vi "Autonomous Independent.vi"() -> ()   [LabVIEW 2014]
doc: "This VI is called when autonomous begins, and will automatically be terminated when autonomous ends. You can carry out timed or sensor driven robot movement independently without needing to return to the caller."
uses:
  <vilib>/Rock Robotics/WPI/Joystick/WPI_JoystickGetSetRefNum.vi
  <vilib>/Rock Robotics/Network Tables/SD Write Numeric Array.vi
  Robot Global Data.vi
  <vilib>/Rock Robotics/WPI/RobotDrive/WPI_RobotDriveGetSetRefNum.vi
  <vilib>/addons/control/pid/pid.llb/PID Advanced (DBL).vi
  <vilib>/Rock Robotics/WPI/RobotDrive/WPI_RobotDriveMecanumDrive_Cartesian.vi
  <vilib>/addons/control/pid/NI_PID_pid.lvlib
panel:
  out "distance":fxp<+/-,32,16>[](array[numeric])
  out "Current Movement, for debugging":T1 {"Z Joystick Value" scale=-1.0..1.0; "Y Joystick Value" scale=1.0..-1.0; "X Joystick Value" scale=-1.0..1.0}
  in  "Array of robot movements":T2(array[cluster]) {"Z Joystick Value" scale=-1.0..1.0; "Y Joystick Value" scale=1.0..-1.0; "X Joystick Value" scale=-1.0..1.0}
  # "Be sure to right-click and choose Data Operations>>Make Current Value default if you want to save the array values with the VI"
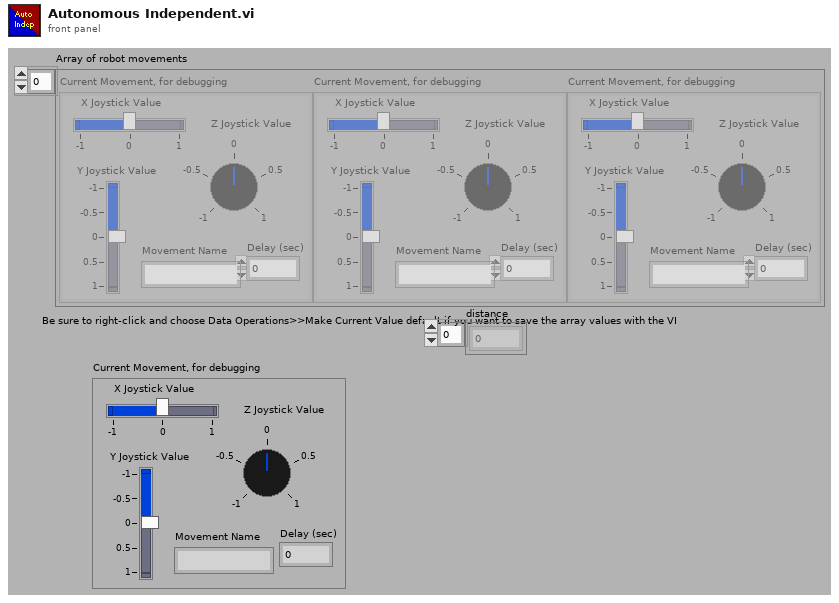
[diagram p1: front panel]
types:
  T1 = cluster{"X Joystick Value":dbl, "Y Joystick Value":dbl, "Z Joystick Value":dbl, "Delay (sec)":dbl, "Movement Name":string}
  T2 = cluster{"X Joystick Value":dbl, "Y Joystick Value":dbl, "Z Joystick Value":dbl, "Delay (sec)":dbl, "Movement Name":string}[]
  T3 = typedef "WPI_EncoderDevRef.ctl" = cluster{"DevStatus":errorcluster, "EncoderIndex":T4, "CounterIndex":T5, "DistancePerCount":dbl, "Decoding Type":T6}
  T4 = typedef "FPGA_EncoderIdx.ctl" = enum8{"Enc 0", "Enc 1", "Enc 2", "Enc 3", "Enc 4", "Enc 5", "Enc 6", "Enc 7", "Invalid"}
  T5 = typedef "FPGA_CounterCtrSystemIndex.ctl" = enum8{"Ctr 0", "Ctr 1", "Ctr 2", "Ctr 3", "Ctr 4", "Ctr 5", "Ctr 6", "Ctr 7", "Invalid"}
  T6 = typedef "WPI_EncoderType.ctl" = enum16{"1x", "2x", "4x"}
  T7 = typedef "WPI_RobotDriveDevRef.ctl" = cluster{"DevStatus":errorcluster, "Motors[]":T8[], "Square Inputs":bool, "Max Output":dbl}
  T8 = typedef "WPI_MotorControlDeviceRef.ctl" = cluster{"DeviceStatus":errorcluster, "Type":T9, "PWM":cluster{"Controller":T10, "PWM Channel":T11, "DeadBand":T12}, "CAN":cluster{"Device Number":u8, "Control Mode":T13, "Semaphore":T14, "Max Vout":dbl, "TalonSRX Control Mode":T15}, "Invert":bool, "TransformRef":T16, "InvTransformRef":T16}
  T9 = typedef "WPI_MotorControlType.ctl" = enum16{"PWM", "CAN", "CANTalonSRX"}
  T10 = typedef "FPGA_TypedefDigitalModule.ctl" = enum16{"Controller 1"}
  T11 = typedef "FPGA_DIOPWMChannel.ctl" = enum8{"PWM 0", "PWM 1", "PWM 2", "PWM 3", "PWM 4", "PWM 5", "PWM 6", "PWM 7", "PWM 8", "PWM 9", "PWM MXP 0", "PWM MXP 1", "PWM MXP 2", "PWM MXP 3", "PWM MXP 4", "PWM MXP 5", "PWM MXP 6", "PWM MXP 7", "PWM MXP 8", "PWM MXP 9", "Invalid"}
  T12 = typedef "WPI_PWMDeadband.ctl" = cluster{"Name":string, "maxPositivePwm":i32, "minPositivePwm":i32, "centerPwm":i32, "maxNegativePwm":i32, "minNegativePwm":i32, "angularRange":u16}
  T13 = typedef "WPI_CANJaguar_ControlMode.ctl" = enum8{"Percent VBus", "Current", "Speed", "Position", "Voltage"}
  T14 = typedef "Semaphore RefNum" = refnum<k1>
  T15 = typedef "WPI_CANTalonSRX_APIControlMode.ctl" = enum8{"Percent VBus", "Speed", "Position", "Slave", "Unchanged / Invalid"}
  T16 = typedef "WPI_PWMTransform_ConPane.ctl" = refnum<vi>
  T17 = typedef "WPI_JoystickDevRef.ctl" = cluster{"Device":T18}
  T18 = typedef "WPI_JoystickDeviceEnum.ctl" = enum16{"USB 0", "USB 1", "USB 2", "USB 3", "USB 4", "USB 5"}
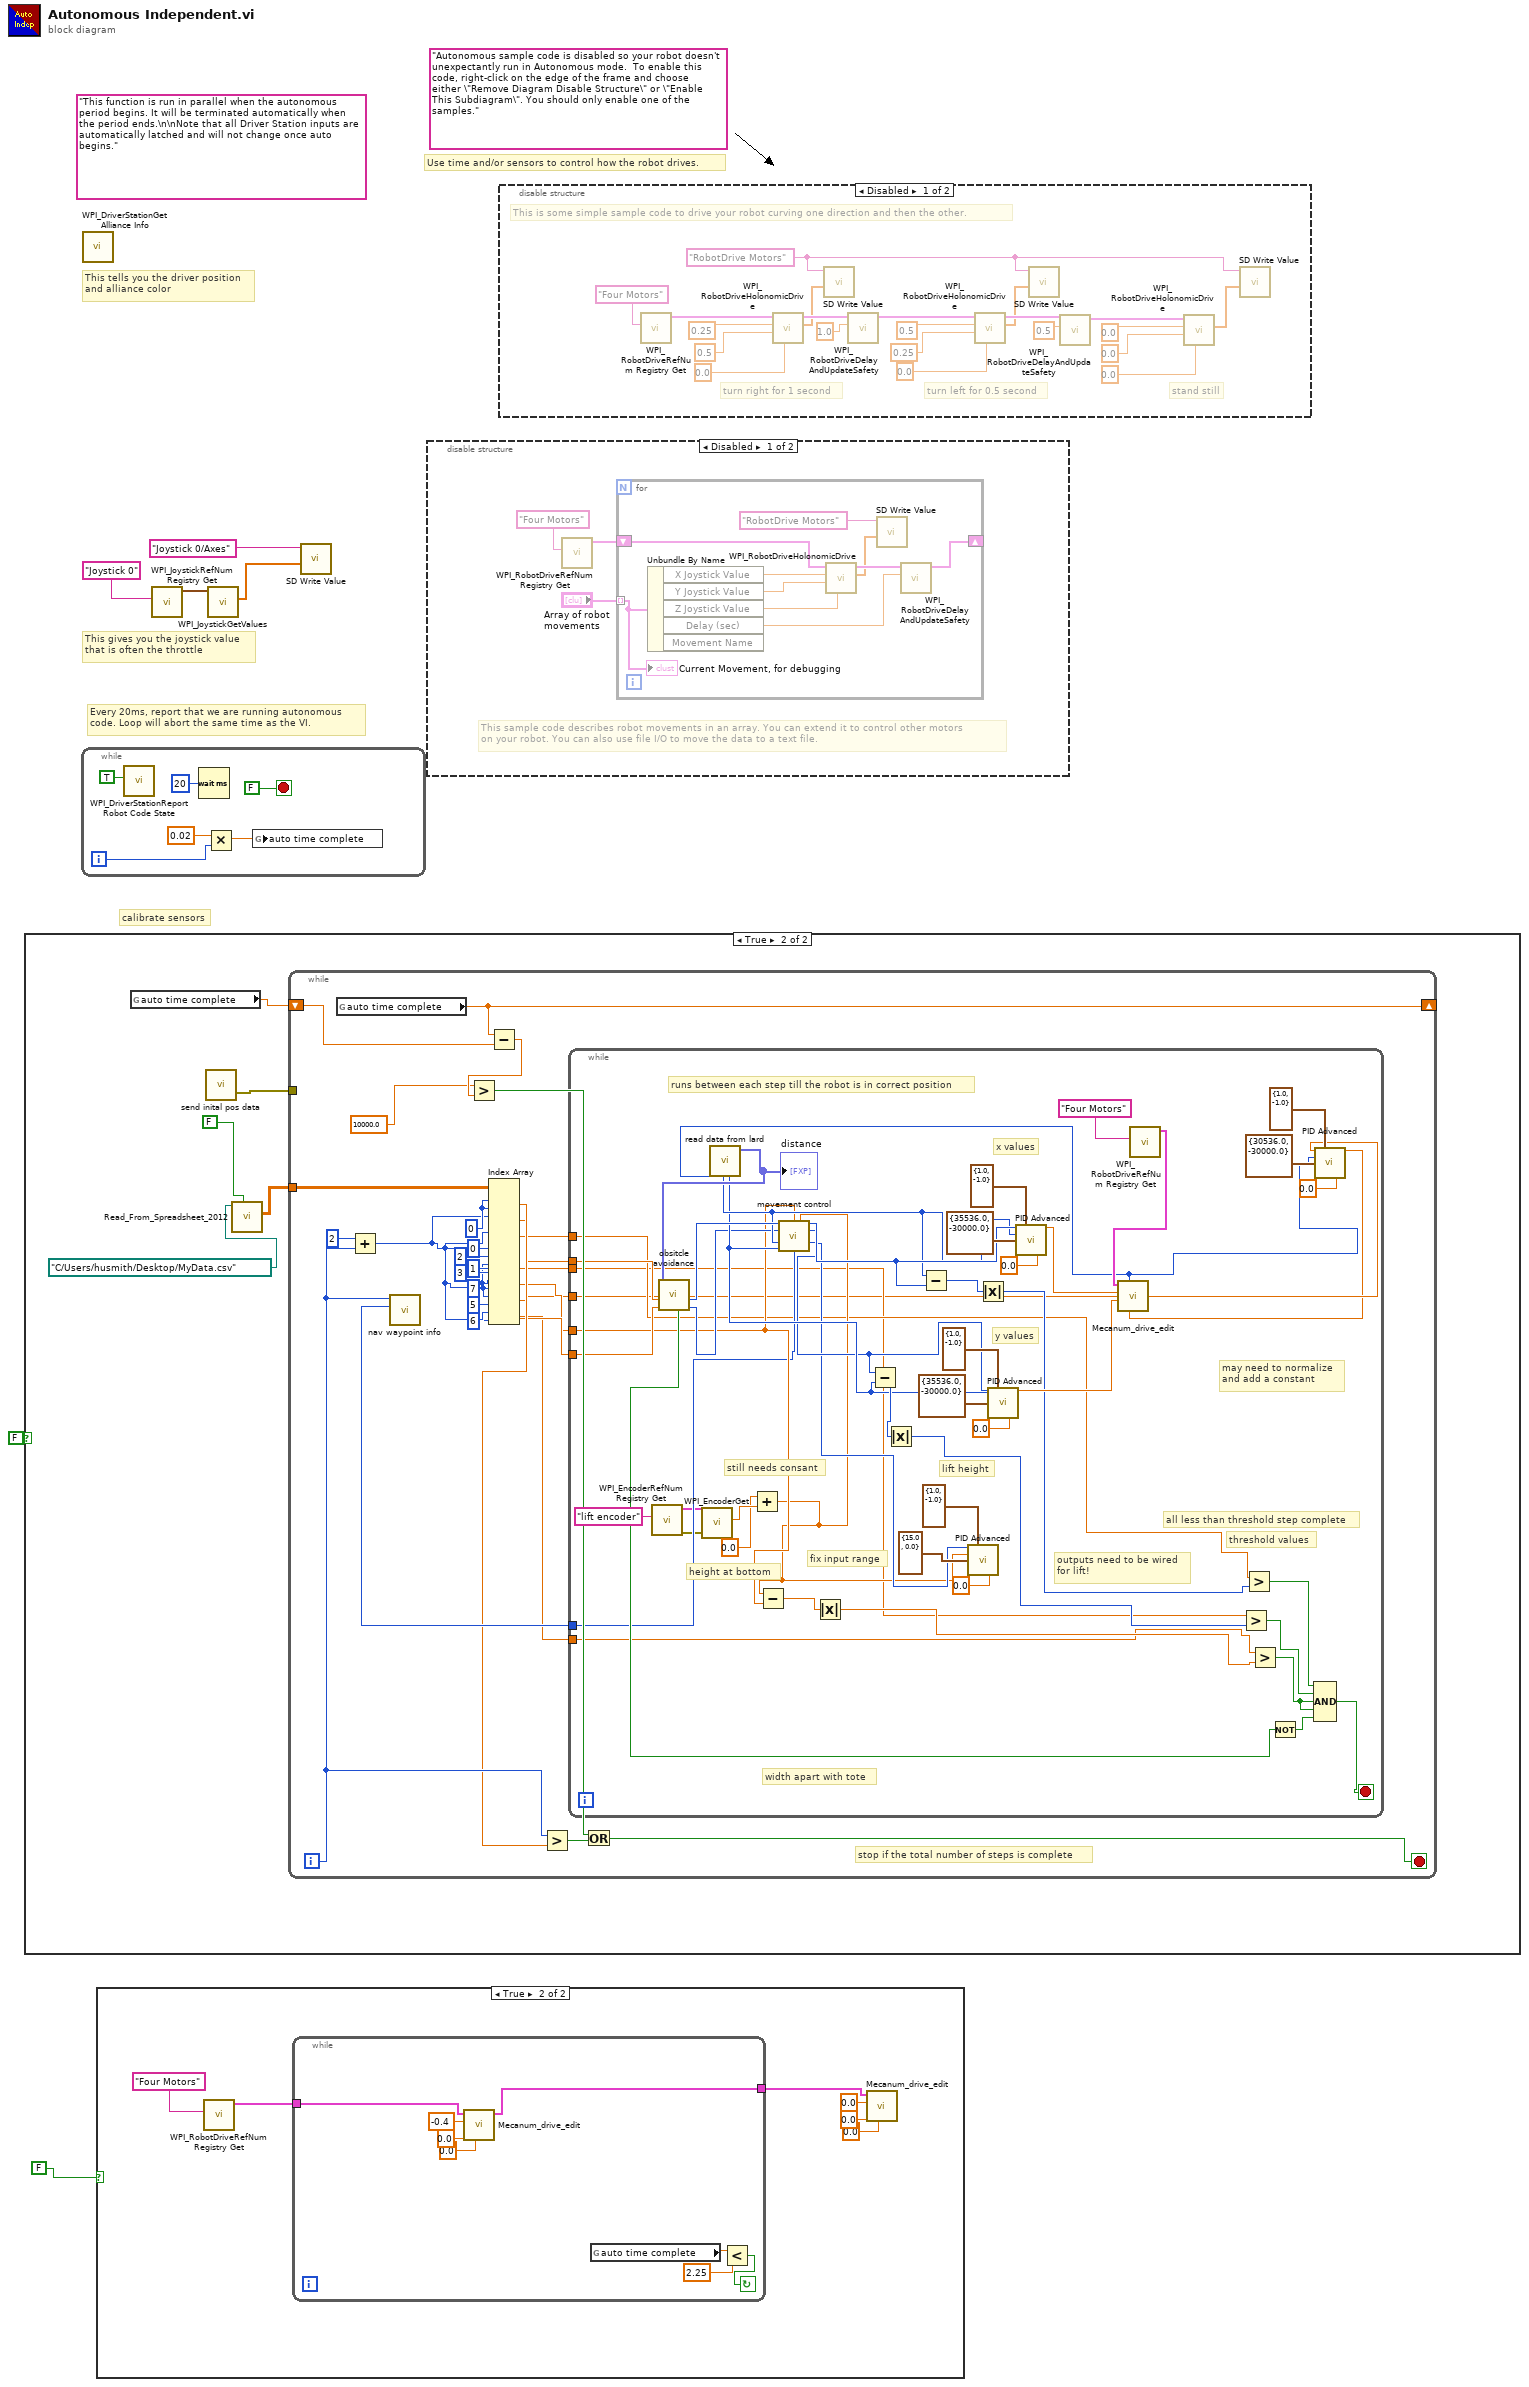
[diagram p0: block diagram]
diagram:
  (unwired) "Autonomous sample code is disabled so your robot doesn't unexpectantly run in Autonomous mode.  To enable this code, right-click on the edge of the frame and choose either \"Remove Diagram Disable Structure\" or \"Enable This Subdiagram\". You should only enable one of the samples."
  (unwired) "This function is run in parallel when the autonomous period begins. It will be terminated automatically when the period ends.\n\nNote that all Driver Station inputs are automatically latched and will not change once auto begins."
  # "calibrate sensors"
  # "Every 20ms, report that we are running autonomous\ncode. Loop will abort the same time as the VI."
  # "This gives you the joystick value\nthat is often the throttle"
  # "Use time and/or sensors to control how the robot drives."
  # "This tells you the driver position\nand alliance color"
  n1 = case shown="True" FALSE {
    frame False {
    }
    frame True {
      n2 = global read "Robot Global Data.vi" "auto time complete"() -> (w11:dbl)
      n3 = call "send inital pos data.vi"() -> ("error out"=w10:errorcluster)  [unwired: 11 in]
      n4 = call "Read_From_Spreadsheet_2012.vi"("My File has Row Headers"=FALSE, "Spreadsheet path (.csv)"=path "C:/Users/husmith/Desktop/MyData.csv") -> ("Data Dsiplay"=w9:dbl[][])  [unwired: 8 in, 1 out]
      n5 = while {
        shift-right: [w38] -> _
        shift-left: w11 -> [w37]
        tunnel: w10 -> [_]
        tunnel: w9 -> [w15]
        i -> [w30]
        stop <- w33 stop-if-true
        w18 = 7 ("disabled index (col)")
        w31 = 0 ("index (row)")
        # "stop if the total number of steps is complete"
        n6 = global read "Robot Global Data.vi" "auto time complete"() -> (w38:dbl)
        n7 = Add(x=2, y=w30) -> (x+y=w14:i32)
        n8 = call "nav waypoint info.vi"("step"=w30) -> ("load"=w39:i32)  [unwired: 6 in, 4 out]
        n9 = Subtract(x=w38, y=w37) -> (x-y=w36:dbl)
        n10 = Greater?(x=10000.0, y=w36) -> (0:w34:bool)
        n11 = Index Array(array=w15, index (row) #1=w31, index (col) #1=w31, index (row) #2=w14, index (col) #2=0 ("disabled index (col)"), index (row) #3=w14, index (col) #3=1 ("disabled index (col)"), index (row) #4=w14, index (col) #4=2 ("disabled index (col)"), index (row) #5=w14, index (col) #5=3 ("disabled index (col)"), index (row) #6=w14, index (col) #6=w18, index (row) #7=w18, index (col) #7=5 ("disabled index (col)"), index (row) #8=w14, index (col) #8=6 ("disabled index (col)")) -> (element #1=w28:dbl, element #2=w26:dbl, element #3=w24:dbl, element #4=w22:dbl, element #5=w20:dbl, element #6=w19:dbl, element #7=w16:dbl, element #8=w12:dbl)
        n12 = Greater?(x=w30, y=w28) -> (0:w35:bool)
        n13 = while {
          tunnel: w26 -> [w69]
          tunnel: w22 -> [w68]
          tunnel: w19 -> [w54]
          tunnel: w39 -> [w52]
          tunnel: w24 -> [w45]
          tunnel: w20 -> [w44]
          tunnel: w16 -> [w43]
          tunnel: w12 -> [w41]
          stop <- w72 stop-if-true
          # "height at bottom"
          # "width apart with tote"
          # "fix input range"
          # "still needs consant"
          # "runs between each step till the robot is in correct position"
          # "outputs need to be wired\nfor lift!"
          # "threshold values"
          # "may need to normalize\nand add a constant"
          # "all less than threshold step complete"
          # "lift height"
          # "y values"
          # "x values"
          n14 = call <vilib>:"WPI_EncoderRefNum Registry Get.vi"("refnum name"="lift encoder") -> ("error out"=w51:errorcluster, "EncoderDevRef"=w50:T3)  [unwired: 9 in]
          n15 = call <vilib>:"WPI_EncoderGet.vi"("error in (no error)"=w51, "EncoderDevRef"=w50) -> ("Distance"=w48:dbl)  [unwired: 4 in, 5 out]
          n16 = call "read data from lard.vi"() -> ("pos x"=w58:i16, "distance"=w61:fxp<+/-,32,16>[], "pos y"=w57:i16, "heading"=w64:i16)  [unwired: 8 in]
          "distance" <- w61
          n17 = call "obsitcle avoidance.vi"("target y"=w68, "target x"=w69, "distance 3"=w61) -> ("target y 2"=w56:i16, "target x 2"=w59:i16, "not done"=w62:bool)  [unwired: 6 in]
          n18 = Add(x=0.0 ("intial position"), y=w48) -> (x+y=w46:dbl)
          n19 = Subtract(x=w46, y=w54) -> (x-y=w76:dbl)
          n20 = call "movement control.vi"("pos x"=w59, "lift"=w54, "current lift"=w46, "pos y"=w56, "current x 2"=w58, "current y 2"=w57, "gripper"=w52) -> ("target x 2"=w60:i16, "target y 2"=w55:i16, "target lift"=w53:i16)  [unwired: 5 in, 1 out]
          n21 = Absolute Value(x=w76) -> (abs(x)=w75:dbl)
          n22 = Subtract(x=w55, y=w57) -> (x-y=w78:i16)
          n23 = Absolute Value(x=w78) -> (abs(x)=w77:i16)
          n24 = Subtract(x=w58, y=w60) -> (x-y=w80:i16)
          n25 = call-poly <vilib>:"PID Advanced.vi"("setpoint"=w53, "output range"=cluster{"output high":dbl, "output low":dbl} {"output high"=1.0, "output low"=-1.0}, "process variable"=w46, "setpoint range"=cluster{"setpoint high":dbl, "setpoint low":dbl} {"setpoint high"=15.0, "setpoint low"=0.0}, "linearity"=0.0) -> ()  [unwired: 9 in, 2 out]
          n26 = Absolute Value(x=w80) -> (abs(x)=w79:i16)
          n27 = call-poly <vilib>:"PID Advanced.vi"("setpoint"=w55, "output range"=cluster{"output high":dbl, "output low":dbl} {"output high"=1.0, "output low"=-1.0}, "process variable"=w57, "setpoint range"=cluster{"setpoint high":dbl, "setpoint low":dbl} {"setpoint high"=35536.0, "setpoint low"=-30000.0}, "linearity"=0.0) -> ("output"=w81:dbl)  [unwired: 9 in, 1 out]
          n28 = call-poly <vilib>:"PID Advanced.vi"("setpoint"=w60, "output range"=cluster{"output high":dbl, "output low":dbl} {"output high"=1.0, "output low"=-1.0}, "process variable"=w58, "setpoint range"=cluster{"setpoint high":dbl, "setpoint low":dbl} {"setpoint high"=35536.0, "setpoint low"=-30000.0}, "linearity"=0.0) -> ("output"=w82:dbl)  [unwired: 9 in, 1 out]
          n29 = call <vilib>:"WPI_RobotDriveRefNum Registry Get.vi"("refnum name"="Four Motors") -> ("RobotDriveDevRef"=w70:T7)  [unwired: 1 in, 9 out]
          n30 = Greater?(x=w44, y=w77) -> (0:w73:bool)
          n31 = Greater?(x=w45, y=w79) -> (0:w74:bool)
          n32 = Greater?(x=w41, y=w75) -> (0:w42:bool)
          n33 = Not(x=w62) -> (.not. x?=w63:bool)
          n34 = Compound Arithmetic op=AND(w74, w73, w42, w42, w63) -> (w72:bool)
          n35 = call-poly <vilib>:"PID Advanced.vi"("setpoint"=w43, "output range"=cluster{"output high":dbl, "output low":dbl} {"output high"=1.0, "output low"=-1.0}, "process variable"=w64, "setpoint range"=cluster{"setpoint high":dbl, "setpoint low":dbl} {"setpoint high"=30536.0, "setpoint low"=-30000.0}, "linearity"=0.0) -> ("output"=w40:dbl)  [unwired: 9 in, 1 out]
          n36 = call "Mecanum_drive_edit.vi"("Rotation"=w40, "Gyro Angle"=w64, "Y"=w81, "X"=w82, "RobotDriveDevRef"=w70) -> ()  [unwired: 4 in, 3 out]
        }
        n37 = Or(x=w34, y=w35) -> (x .or. y?=w33:bool)
      }
    }
  }
  n38 = while {
    i -> [w93]
    stop <- FALSE stop-if-true
    n39 = call <vilib>:"WPI_DriverStationReport Robot Code State.vi"("Autonomous"=TRUE) -> ()  [unwired: 10 in, 1 out]
    n40 = Wait (ms)(milliseconds to wait=u32 20) -> ()  [unwired: 1 out]
    n41 = Multiply(x=0.02, y=w93) -> (x*y=w92:dbl)
    n42 = global write "Robot Global Data.vi" "auto time complete"(w92) -> ()
  }
  n43 = call <vilib>:"WPI_DriverStationGet Alliance Info.vi"() -> ()  [unwired: 12 out]
  n44 = case shown="True" FALSE {
    frame False {
    }
    frame True {
      n45 = call <vilib>:"WPI_RobotDriveRefNum Registry Get.vi"("refnum name"="Four Motors") -> ("RobotDriveDevRef"=w102:T7)  [unwired: 1 in, 9 out]
      n46 = while {
        tunnel: w102 -> [w105]
        tunnel: [w104] -> w98
        stop <- w111 continue-if-true
        n47 = call "Mecanum_drive_edit.vi"("Rotation"=0.0, "Y"=0.0, "X"=-0.4, "RobotDriveDevRef"=w105) -> ("RobotDriveDevRef"=w104:T7)  [unwired: 5 in, 2 out]
        n48 = global read "Robot Global Data.vi" "auto time complete"() -> (w110:dbl)
        n49 = Less?(x=w110, y=2.25) -> (x < y?=w111:bool)
      }
      n50 = call "Mecanum_drive_edit.vi"("Rotation"=0.0, "Y"=0.0, "X"=0.0, "RobotDriveDevRef"=w98) -> ()  [unwired: 5 in, 3 out]
    }
  }
  n51 = call <vilib>:"WPI_JoystickRefNum Registry Get.vi"("refnum name"="Joystick 0") -> ("JoystickDevRef"=w5:T17)  [unwired: 1 in, 9 out]
  n52 = call <vilib>:"WPI_JoystickGetValues.vi"("JoystickDevRef"=w5) -> ("Axes"=w3:dbl[])  [unwired: 6 in, 4 out]
  n53 = call-poly <vilib>:"SD Write Value.vi"("Numeric Array"=w3, "Name"="Joystick 0/Axes") -> ()  [unwired: 8 in, 2 out]
  n54 = disable-structure shown="Disabled" {
    frame Disabled {
      # "This sample code describes robot movements in an array. You can extend it to control other motors\non your robot. You can also use file I/O to move the data to a text file."
      n55 = call <vilib>:"WPI_RobotDriveRefNum Registry Get.vi"("refnum name"="Four Motors") -> ("RobotDriveDevRef"=w113:T7)  [unwired: 1 in, 9 out]
      n56 = for {
        shift-right: [w121] -> _
        shift-left: w113 -> [w122]
        tunnel: "Array of robot movements" -> [w117] mode=indexing
        n57 = Unbundle By Name(w117) -> ("X Joystick Value"=w120:dbl, "Y Joystick Value"=w119:dbl, "Z Joystick Value"=w116:dbl, "Delay (sec)"=w118:dbl)  [unwired: 1 out]
        n58 = call-poly <vilib>:"WPI_RobotDriveHolonomicDrive.vi"("Rotation"=w116, "Y"=w119, "X"=w120, "RobotDriveDevRef"=w122) -> ("Motor Values"=w115:dbl[], "RobotDriveDevRef"=w123:T7)  [unwired: 5 in, 1 out]
        n59 = call-poly <vilib>:"SD Write Value.vi"("Numeric Array"=w115, "Name"="RobotDrive Motors") -> ()  [unwired: 8 in, 2 out]
        n60 = call <vilib>:"WPI_RobotDriveDelayAndUpdateSafety.vi"("Delay (s)"=w118, "RobotDriveDevRef"=w123) -> ("RobotDriveDevRef 2"=w121:T7)  [unwired: 8 in, 1 out]
        "Current Movement, for debugging" <- w117
      }
    }
    frame Enabled {
    }
  }
  n61 = disable-structure shown="Disabled" {
    frame Disabled {
      w131 = "RobotDrive Motors" ("Name")
      # "This is some simple sample code to drive your robot curving one direction and then the other."
      # "stand still"
      # "turn left for 0.5 second"
      # "turn right for 1 second"
      n62 = call <vilib>:"WPI_RobotDriveRefNum Registry Get.vi"("refnum name"="Four Motors") -> ("RobotDriveDevRef"=w132:T7)  [unwired: 1 in, 9 out]
      n63 = call-poly <vilib>:"WPI_RobotDriveHolonomicDrive.vi"("Rotation"=0.0, "Y"=0.5 ("X axis value"), "X"=0.25 ("X axis value"), "RobotDriveDevRef"=w132) -> ("Motor Values"=w127:dbl[], "RobotDriveDevRef"=w139:T7)  [unwired: 5 in, 1 out]
      n64 = call-poly <vilib>:"SD Write Value.vi"("Numeric Array"=w127, "Name"=w131) -> ()  [unwired: 8 in, 2 out]
      n65 = call <vilib>:"WPI_RobotDriveDelayAndUpdateSafety.vi"("Delay (s)"=1.0, "RobotDriveDevRef"=w139) -> ("RobotDriveDevRef 2"=w138:T7)  [unwired: 8 in, 1 out]
      n66 = call-poly <vilib>:"WPI_RobotDriveHolonomicDrive.vi"("Rotation"=0.0, "Y"=0.25 ("X axis value"), "X"=0.5 ("X axis value"), "RobotDriveDevRef"=w138) -> ("Motor Values"=w126:dbl[], "RobotDriveDevRef"=w137:T7)  [unwired: 5 in, 1 out]
      n67 = call-poly <vilib>:"SD Write Value.vi"("Numeric Array"=w126, "Name"=w131) -> ()  [unwired: 8 in, 2 out]
      n68 = call <vilib>:"WPI_RobotDriveDelayAndUpdateSafety.vi"("Delay (s)"=0.5, "RobotDriveDevRef"=w137) -> ("RobotDriveDevRef 2"=w136:T7)  [unwired: 8 in, 1 out]
      n69 = call-poly <vilib>:"WPI_RobotDriveHolonomicDrive.vi"("Rotation"=0.0 ("X axis value"), "Y"=0.0 ("X axis value"), "X"=0.0 ("X axis value"), "RobotDriveDevRef"=w136) -> ("Motor Values"=w125:dbl[])  [unwired: 5 in, 2 out]
      n70 = call-poly <vilib>:"SD Write Value.vi"("Numeric Array"=w125, "Name"=w131) -> ()  [unwired: 8 in, 2 out]
    }
    frame Enabled {
    }
  }
